vi "split_error.vi"(8 "error in":errorcluster) -> (0 "error out":errorcluster, 1 "callStack":string, 2 "Location":string, 3 "Details":string)   [LabVIEW 2020]
uses:
  <vilib>/ErrorRing/Error Ring.xnode
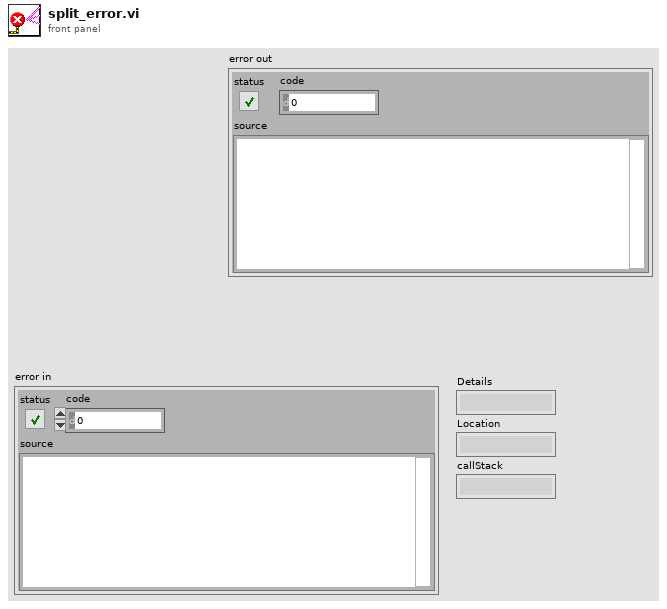
[diagram p1: front panel]
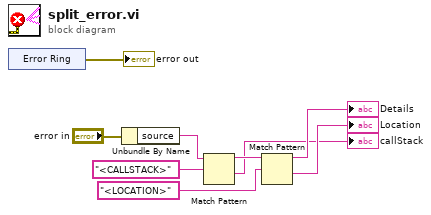
[diagram p0: block diagram]
diagram:
  n1 = xnode "Error Ring"() -> ("error out"=→"error out":errorcluster)
  n2 = Unbundle By Name("error in") -> ("source"=w8:string)
  n3 = Match Pattern(string=w8, regular expression="<CALLSTACK>" ("string")) -> (before substring=w4:string, after substring=→"callStack":string)  [unwired: 1 in, 2 out]
  n4 = Match Pattern(string=w4, regular expression="<LOCATION>" ("string")) -> (before substring=→"Details":string, after substring=→"Location":string)  [unwired: 1 in, 2 out]
